vi "Write Bin.vi"(8 "Error In":errorcluster) -> (0 "Error Out":errorcluster)   [LabVIEW 2017, in "Tests.lvlib" / "Writer.lvlib"]
uses:
  Writer.lvlib
  src/LabPack/Public/Writer/Writer.lvclass/Writer.ctl
  src/LabPack/Public/Writer/Private/Handle Error.vi
  src/LabPack/Public/Writer/Public/Status/Read Is Error.vi
  src/LabPack/Public/Writer/Public/Status/Read Status.vi
  src/LabPack/Public/Writer/Public/Status/Read Status Message.vi
  src/LabPack/Public/Utility/Status Code.vi
  <vilib>/Utility/error.llb/Error Cluster From Error Code.vi
  <vilib>/addons/_JKI Toolkits/Caraya/classes/Test/Test.lvclass
  <vilib>/addons/_JKI Toolkits/Caraya/classes/Assert/Assert.lvclass
  src/LabPack/Public/Writer/Writer.lvclass
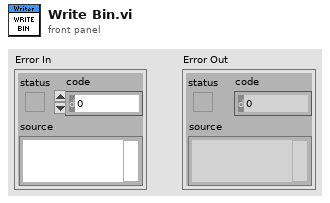
[diagram p1: front panel]
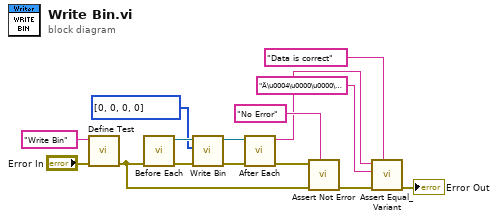
[diagram p0: block diagram]
diagram:
  n1 = call <vilib>:"Define Test.vi"("error in (no error)"="Error In", "Label (VI Title)"="Write Bin") -> ("error out"=w11:errorcluster)  [unwired: 9 in]
  n2 = call "Before Each.vi"("Error In"=w11) -> ("Error Out"=w7:errorcluster, "Writer Out"=w6:refnum<class "Writer.lvclass">)  [unwired: 9 in]
  n3 = call "Write Bin.vi"("Error In"=w7, "Value"=u8[] [0, 0, 0, 0], "Writer In"=w6) -> ("Error Out"=w4:errorcluster, "Writer Out"=w5:refnum<class "Writer.lvclass">)  [unwired: 7 in]
  n4 = call "After Each.vi"("Error In"=w4, "Writer In"=w5) -> ("Error Out"=w10:errorcluster, "Data"=w3:string)  [unwired: 8 in]
  n5 = call <vilib>:"Assert Not Error.vi"("Label"="No Error", "error in (no error)"=w11, "Not Error?"=w10) -> ("error out"=w13:errorcluster)  [unwired: 8 in]
  n6 = call <vilib>:"Assert Equal_Variant.vi"("Label"="Data is correct", "error in (no error)"=w13, "Y"="Ä\u0004\u0000\u0000\u0000\u0000" ("Data"), "X"=w3) -> ("error out"=→"Error Out":errorcluster)  [unwired: 7 in]
